vi "CRYGet Interpolation MinMax.vi"(4 "Fu":dbl[](array[numeric]), 6 "Fl":dbl[](array[numeric]), 8 "y":dbl[](array[numeric]), 9 "x":dbl[](array[numeric])) -> (3 "y":dbl[](array[numeric]))   [LabVIEW 2013]
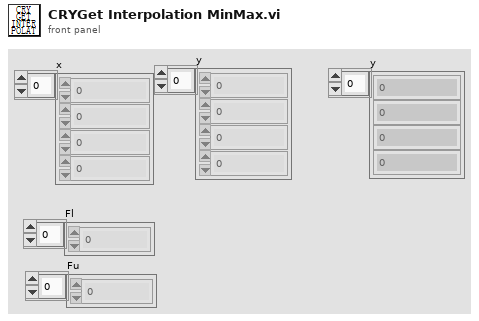
[diagram p1: front panel]
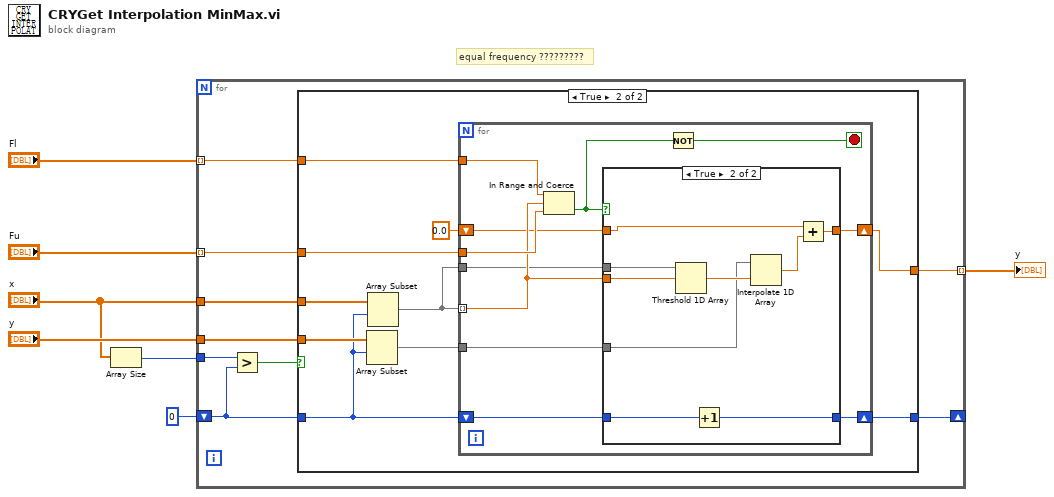
[diagram p0: block diagram]
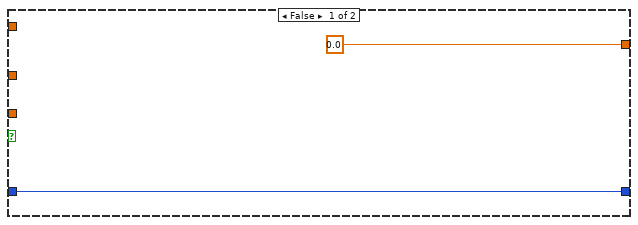
[diagram p2: hidden frame]
diagram:
  # "equal frequency ?????????"
  n1 = Array Size(array="x") -> (size(s)=w1:i32)
  n2 = for {
    tunnel: [w16] -> w6 mode=indexing
    tunnel: "y" -> [w15]
    tunnel: "x" -> [w12]
    tunnel: "Fl" -> [w14] mode=indexing
    tunnel: "Fu" -> [w13] mode=indexing
    tunnel: w1 -> [w11]
    shift-right: [w8] -> _
    shift-left: 0 -> [w10]
    n3 = Greater?(x=w11, y=w10) -> (0:w9:bool)
    n4 = case shown="True" w9 {
      tunnel: [0.0 ("fractional index or x") w19] -> w16
      tunnel: w15 -> [_ w22]
      tunnel: w14 -> [_ w28]
      tunnel: w13 -> [_ w27]
      tunnel: w12 -> [_ w25]
      tunnel: w10 -> [w17 w21]
      tunnel: [w17 w26] -> w8
      frame False {
      }
      frame True {
        n5 = Array Subset(array=w22, index=w21) -> (w20:dbl[])  [unwired: 1 in]
        n6 = Array Subset(array=w25, index=w21) -> (w24:dbl[])  [unwired: 1 in]
        n7 = for {
          tunnel: w20 -> [w39]
          tunnel: w28 -> [w38]
          tunnel: w27 -> [w37]
          tunnel: w24 -> [w36] mode=indexing
          tunnel: w24 -> [w33]
          shift-right: [w35] -> w26
          shift-left: w21 -> [w34]
          shift-right: [w30] -> w19
          shift-left: 0.0 ("fractional index or x") -> [w29]
          stop <- w31 stop-if-true
          n8 = In Range and Coerce(upper limit=w38, x=w36, lower limit=w37) -> (In Range?=w32:bool)  [unwired: 1 out]
          n9 = case shown="True" w32 {
            tunnel: w36 -> [_ w50]
            tunnel: w39 -> [_ w48]
            tunnel: [w41 w46] -> w35
            tunnel: w34 -> [w41 w47]
            tunnel: w33 -> [_ w45]
            tunnel: [w40 w42] -> w30
            tunnel: w29 -> [w40 w44]
            frame False {
            }
            frame True {
              n10 = Threshold 1D Array(2:w50, 3:w45) -> (0:w49:dbl)  [unwired: 1 in]
              n11 = Increment(x=w47) -> (x+1=w46:i32)
              n12 = Interpolate 1D Array(1:w49, 2:w48) -> (0:w43:dbl)
              n13 = Add(x=w44, y=w43) -> (x+y=w42:dbl)
            }
          }
          n14 = Not(x=w32) -> (.not. x?=w31:bool)
        }
      }
    }
  }
  "y" <- w6
